vi "Data Acquisition.vi"(8 "Reset?":bool) -> (0 "Data Packet":T1)   [LabVIEW 2015]
uses:
  Drivetrain Data AQ Packet.ctl
  navX-MXP Library/COMMON/TypeDefs/Data TypeDefs/navX Vector Data.ctl
  <vilib>/Utility/file.llb/Write Delimited Spreadsheet (DBL).vi
  navX-MXP Library/navX-MXP IMU.lvlib
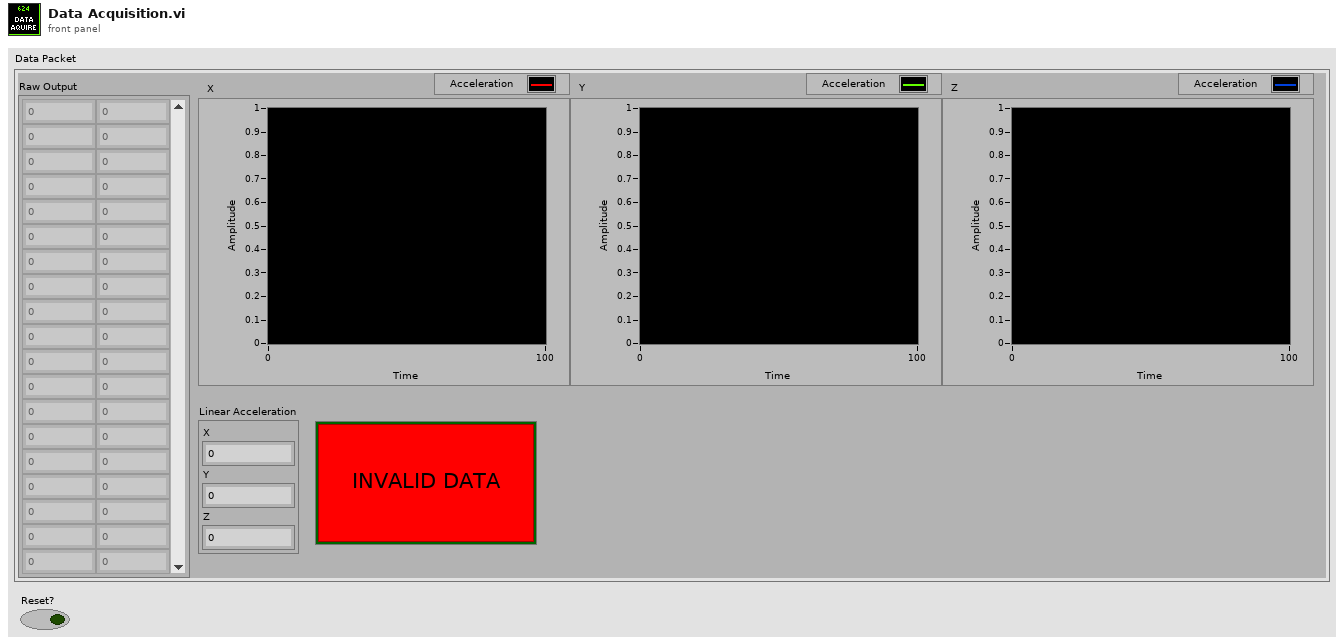
[diagram p1: front panel]
types:
  T1 = typedef "Drivetrain Data AQ Packet.ctl" = cluster{"Linear Acceleration":T2, "Raw Output":dbl[][], "X":dbl, "Y":dbl, "Z":dbl, "Valid?":bool}
  T2 = typedef "navX-MXP IMU.lvlib/navX Vector Data.ctl" = cluster{"X":dbl, "Y":dbl, "Z":dbl}
  T3 = typedef "navX-MXP IMU.lvlib/navX Device TypeDef.ctl" = cluster{"navX Interface Protocol":T4, "navX Interface Protocol TypeDefs":cluster{"SPIDevRef":T5, "I2CDevRef":T7}, "navX System Information":cluster{"Board Information":T9, "Status":T10, "Offsets":T14}, "navX Common Information":cluster{"Update Rate (4Hz-60Hz)":T15, "refnum name":string, "error":errorcluster}}
  T4 = typedef "navX-MXP IMU.lvlib/navX Interface Protocol.ctl" = enum16{"SPI", "I2C"}
  T5 = typedef "WPI_SPIDevRef.ctl" = cluster{"DevStatus":errorcluster, "Handle":i32, "SPI Bus":T6}
  T6 = typedef "spi_bus.ctl" = enum16{"SPI On-Board, CS0", "SPI On-Board, CS1", "SPI On-Board, CS2", "SPI On-Board, CS3", "SPI MXP", "Invalid"}
  T7 = typedef "WPI_I2CDevRef.ctl" = cluster{"DevStatus":errorcluster, "Device Address":u8, "Handle":i32, "I2C Bus":T8}
  T8 = typedef "i2c_bus.ctl" = enum16{"I2C On-Board", "I2C MXP", "Invalid"}
  T9 = typedef "navX-MXP IMU.lvlib/navX Board Information.ctl" = cluster{"WhoAmI (50 | 0x32)":u8, "Board Revision":u8, "Firmware Major Version":u8, "Firmware Minor Version":u8}
  T10 = typedef "navX-MXP IMU.lvlib/navX Status Data.ctl" = cluster{"Update Rate Hz":u8, "Accelerometer Full-Scale Range":u8, "Gyro Full-Scale Range":u16, "NAVX_OP_STATUS":T11, "NAVX_CAL_STATUS":T12, "NAVX_SELFTEST_STATUS":u8, "NAVX_SENSOR_STATUS":T13}
  T11 = typedef "navX-MXP IMU.lvlib/navX NAVX_OP_STATUS.ctl" = u8
  T12 = typedef "navX-MXP IMU.lvlib/navX NAVX_CAL_STATUS.ctl" = u8
  T13 = typedef "navX-MXP IMU.lvlib/navX NAVX_SENSOR_STATUS.ctl" = cluster{"MOVING":bool, "YAW_STABLE":bool, "MAG_DISTURBANCE":bool, "ALTITUDE_VALID":bool, "SEALEVEL_PRESS_SET":bool, "FUSED_HEADING_VALID":bool}
  T14 = typedef "navX-MXP IMU.lvlib/navX Offsets Data.ctl" = cluster{"Yaw":dbl, "Quat W":dbl, "Quat X":dbl, "Quat Y":dbl, "Quat Z":dbl}
  T15 = typedef "navX-MXP IMU.lvlib/navX Update Rate.ctl" = u8
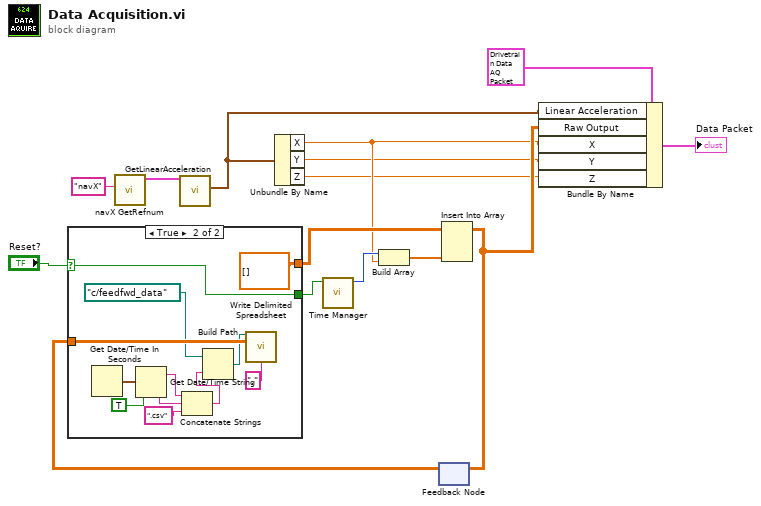
[diagram p0: block diagram]
diagram:
  n1 = call "navX GetRefnum.vi"("refnum name"="navX") -> ("navX Device TypeDef"=w9:T3)  [unwired: 9 in, 1 out]
  n2 = call "GetLinearAcceleration.vi"("navX Device TypeDef"=w9) -> ("Linear Acceleration"=w6:T2)  [unwired: 8 in, 2 out]
  n3 = Unbundle By Name(w6) -> ("X"=w4:dbl, "Y"=w3:dbl, "Z"=w2:dbl)
  n4 = feedback #1() -> (w14:dbl[][])  [unwired: 1 in]
  n5 = case shown="True" "Reset?" {
    selector: "Reset?" -> [w16 w28]
    tunnel: [w17 dbl[][] []] -> w15
    tunnel: w14 -> [w17 w27]
    tunnel: [w16 w28] -> w12
    frame False {
    }
    frame True {
      n6 = Get Date/Time In Seconds() -> (seconds since 1Jan1904=w24:timestamp)
      n7 = Get Date/Time String(seconds (now)=w24, want seconds? (F)=TRUE) -> (date string=w22:string, time string=w21:string)  [unwired: 1 in]
      n8 = Concatenate Strings(w22, w21, ".csv" ("string")) -> (w20:string)
      n9 = Build Path(base path=path "c/feedfwd_data", name or relative path=w20) -> (appended path=w26:path)
      n10 = call-poly <vilib>:"Write Delimited Spreadsheet.vi"("file path (dialog if empty)"=w26, "2D data"=w27, "delimiter (\\t)"="," ("delimiter (\\t)")) -> ()  [unwired: 11 in, 2 out]
    }
  }
  n11 = call "Time Manager.vi"("Reset?"=w12) -> ("Elapsed Time"=w11:u32)  [unwired: 10 in]
  n12 = Build Array(w11, w4) -> (w10:dbl[])
  n13 = Insert Into Array(array=w15, new element=w10) -> (w5:dbl[][])  [unwired: 2 in]
  n14 = feedback-in #1(w5) -> ()
  n15 = Bundle By Name(cluster=T1 {"Linear Acceleration"={"X"=0.0, "Y"=0.0, "Z"=0.0}, "Raw Output"=[], "X"=0.0, "Y"=0.0, "Z"=0.0, "Valid?"=FALSE} ("Data Packet"), "Linear Acceleration"=w6, "Raw Output"=w5, "X"=w4, "Y"=w3, "Z"=w2) -> (→"Data Packet":T1)
